vi "GenPolice.vi"(5 "Color 2":u32(colorbox)=16860, 6 "Reset":bool, 7 "Color 1":u32(colorbox)=16711680, 10 "Period":i32=200, 11 "NumLeds":i32) -> (3 "Array":u32[](array[numeric]))   [LabVIEW 2023, in "ArduinoSerialBling.lvlib"]
uses:
  ArduinoSerialBling.lvlib
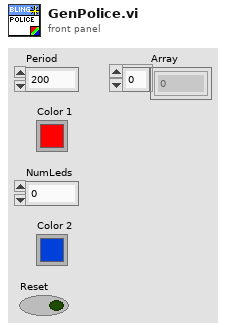
[diagram p1: front panel]
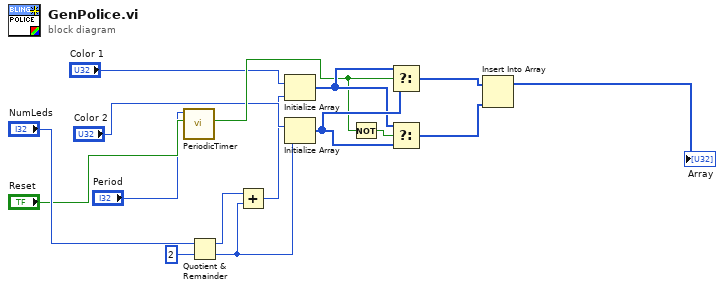
[diagram p0: block diagram]
diagram:
  n1 = call "PeriodicTimer.vi"("Reset"="Reset", "Period (ms)"="Period") -> ("Square Wave"=w11:bool)  [unwired: 7 in, 2 out]
  n2 = Quotient & Remainder(x="NumLeds", y=2) -> (x-y*floor(x/y)=w5:i32, floor(x/y)=w7:i32)
  n3 = Add(x=w5, y=w7) -> (x+y=w6:i32)
  n4 = Initialize Array("Color 1", w6) -> (w12:u32[])
  n5 = Initialize Array("Color 2", w7) -> (w13:u32[])
  n6 = Not(x=w11) -> (.not. x?=w10:bool)
  n7 = Select(t=w12, s=w11, f=w13) -> (s? t:f=w14:u32[])
  n8 = Select(t=w12, s=w10, f=w13) -> (s? t:f=w15:u32[])
  n9 = Insert Into Array(array=w14, new element=w15) -> (→"Array":u32[])  [unwired: 1 in]
